vi "SendCMD&ReadValue.vi"() -> ()   [LabVIEW 2017, in "4040.lvlib"]
uses:
  4040.lvlib
  CommandType.ctl
panel:
  out "DataOut":variant
  in  "DataIn":variant
  in  "CommandType":T1
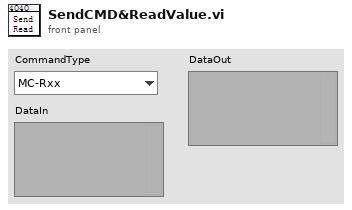
[diagram p1: front panel]
types:
  T1 = typedef "4040.lvlib/CommandType.ctl" = enum16{"MC-Rxx", "MC-Save", "MC-Default", "MC-SN", "MC-MN", "MC-Rev", "MC-Date", "MC-?", "DC-Surnnnn", "DC-SDMm", "DC-SDMFTPn", "DC-SDUn"}
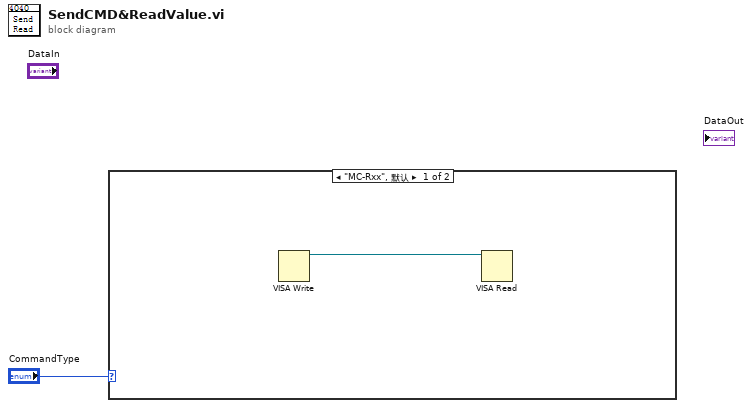
[diagram p0: block diagram]
diagram:
  n1 = case shown="\"MC-Rxx\", 默认" "CommandType" {
    frame "MC-Rxx", Default {
      n2 = VISA Write() -> (VISA resource name out=w2:refnum<visa-resource-name>)  [unwired: 3 in, 2 out]
      n3 = VISA Read(VISA resource name=w2) -> ()  [unwired: 2 in, 4 out]
    }
    frame "MC-Save" {
    }
  }
